vi "main.vi"   [LabVIEW 2013]
doc: "Use this template to build a standard state machine design pattern. Each state executes code and determines which state to transition to. Contrast this design pattern with the User Interface Event Handler pattern, in which code executes in response to user actions. Contrast this design pattern also with the Queued Message Handler pattern, in which each message handling code can queue zero or more new messages.\nNote: This template does not contain the most recent programming guidelines recommended by National Instruments. For a complete, project-based implementation of the Standard State Machine pattern, use the Create Project dialog box instead of this template."
uses:
  StateMachineStates.ctl
types:
  T1 = typedef "StateMachineStates.ctl" = enum16{"Initialize", "Idle", "Calibration", "Aux Correction", "Take Measurement", "Notify Operator", "Stop"}
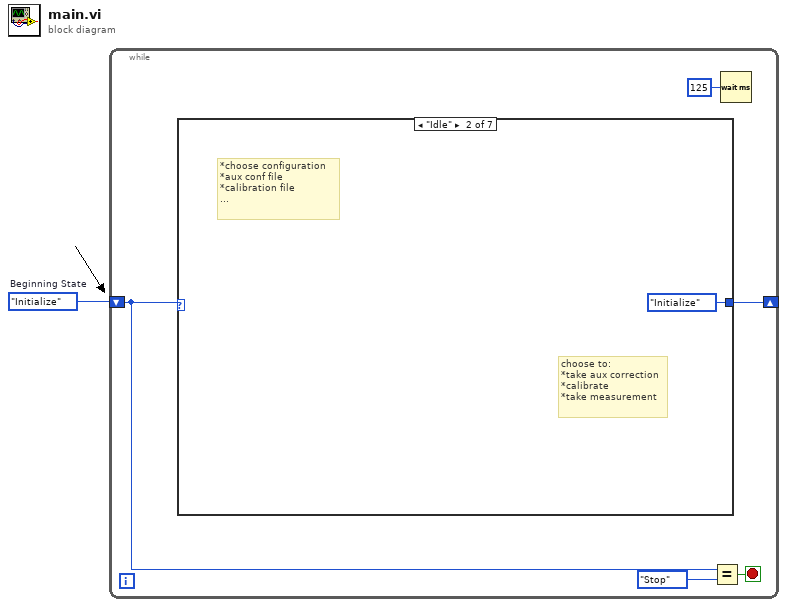
[diagram p0: block diagram]
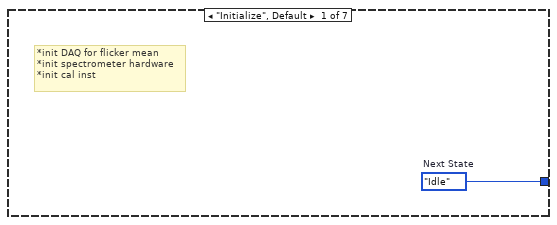
[diagram p2: hidden frame]
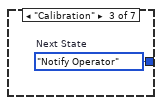
[diagram p3: hidden frame]
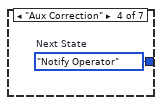
[diagram p4: hidden frame]
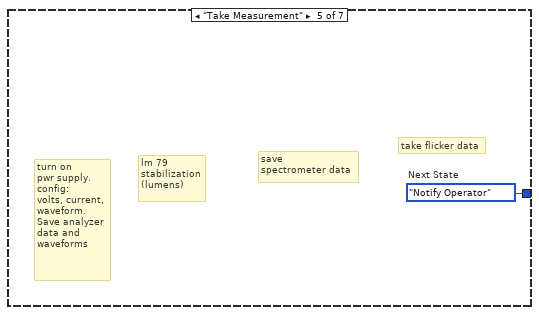
[diagram p5: hidden frame]
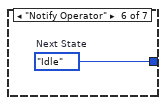
[diagram p6: hidden frame]
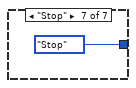
[diagram p7: hidden frame]
diagram:
  w1 = StateMachineStates."Initialize"  # Beginning State
  n1 = while {
    shift-right: [w3] -> _
    shift-left: w1 -> [w4]
    stop <- w6 stop-if-true
    n2 = case shown="\"Idle\"" w4 {
      tunnel: [w7 StateMachineStates."Initialize" ("Next State") w9 w10 w11 w12 StateMachineStates."Stop" ("Next State")] -> w3
      frame "Initialize", Default {
        w7 = StateMachineStates."Idle"  # Next State
        # "*init DAQ for flicker mean\n*init spectrometer hardware\n*init cal inst"
      }
      frame "Idle" {
        # "choose to:\n*take aux correction\n*calibrate\n*take measurement"
        # "*choose configuration\n*aux conf file\n*calibration file\n..."
      }
      frame "Calibration" {
        w9 = StateMachineStates."Notify Operator"  # Next State
      }
      frame "Aux Correction" {
        w10 = StateMachineStates."Notify Operator"  # Next State
      }
      frame "Take Measurement" {
        w11 = StateMachineStates."Notify Operator"  # Next State
        # "take flicker data"
        # "save\nspectrometer data"
        # "lm 79 \nstabilization\n(lumens)"
        # "turn on\npwr supply.\nconfig:\nvolts, current,\nwaveform. \nSave analyzer\ndata and\nwaveforms"
      }
      frame "Notify Operator" {
        w12 = StateMachineStates."Idle"  # Next State
      }
      frame "Stop" {
      }
    }
    n3 = Equal?(x=w4, y=StateMachineStates."Stop" ("States")) -> (x = y?=w6:bool)
    n4 = Wait (ms)(milliseconds to wait=u32 125) -> ()  [unwired: 1 out]
  }
